vi "Helper SubVI - Fusion Method.vi"(6 "method":u16(ring)=2 items=["Max", "Min", "Mean", "Image 1", "Image 2"], 9 "Coef 2":i32[][](array[numeric]), 11 "Coef 1":i32[][](array[numeric])) -> (3 "Fusion Coef":i32[][](array[numeric]))   [LabVIEW 2023]
doc: "Merges the input coefficients."
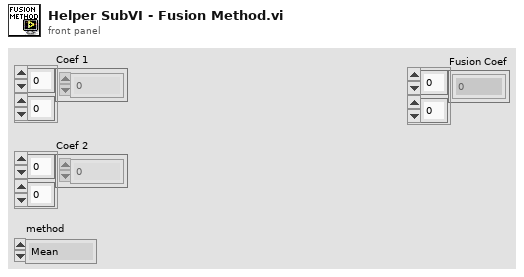
[diagram p1: front panel]
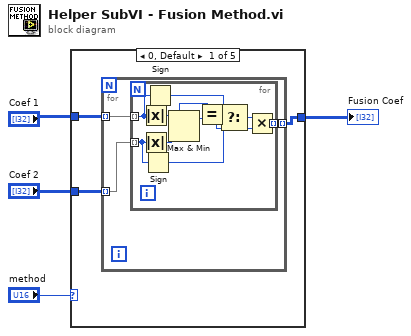
[diagram p0: block diagram]
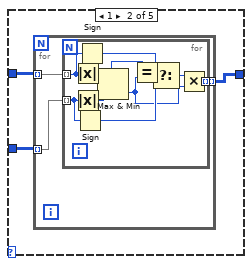
[diagram p2: hidden frame]
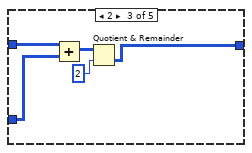
[diagram p3: hidden frame]
diagram:
  n1 = case shown="0, Default" "method" {
    tunnel: "Coef 1" -> [w7 w23 w41 w42 _]
    tunnel: "Coef 2" -> [w6 w22 w40 _ w43]
    tunnel: [w5 w21 w37 w42 w43] -> w1
    frame 0, Default {
      n2 = for {
        tunnel: w7 -> [w10] mode=indexing
        tunnel: w6 -> [w9] mode=indexing
        tunnel: [w8] -> w5 mode=indexing
        n3 = for {
          tunnel: w10 -> [w18] mode=indexing
          tunnel: w9 -> [w19] mode=indexing
          tunnel: [w11] -> w8 mode=indexing
          n4 = Absolute Value(x=w18) -> (abs(x)=w17:i32)
          n5 = Absolute Value(x=w19) -> (abs(x)=w20:i32)
          n6 = Sign(1:w19) -> (0:w14:i32)
          n7 = Sign(1:w18) -> (0:w15:i32)
          n8 = Max & Min(x=w17, y=w20) -> (max(x,y)=w12:i32)  [unwired: 1 out]
          n9 = Equal?(x=w17, y=w12) -> (x = y?=w16:bool)
          n10 = Select(t=w15, s=w16, f=w14) -> (s? t:f=w13:i32)
          n11 = Multiply(x=w13, y=w12) -> (x*y=w11:i32)
        }
      }
    }
    frame 1 {
      n12 = for {
        tunnel: w23 -> [w26] mode=indexing
        tunnel: w22 -> [w25] mode=indexing
        tunnel: [w24] -> w21 mode=indexing
        n13 = for {
          tunnel: w26 -> [w34] mode=indexing
          tunnel: w25 -> [w35] mode=indexing
          tunnel: [w28] -> w24 mode=indexing
          n14 = Absolute Value(x=w34) -> (abs(x)=w33:i32)
          n15 = Absolute Value(x=w35) -> (abs(x)=w36:i32)
          n16 = Sign(1:w35) -> (0:w30:i32)
          n17 = Sign(1:w34) -> (0:w31:i32)
          n18 = Max & Min(x=w33, y=w36) -> (min(x,y)=w27:i32)  [unwired: 1 out]
          n19 = Equal?(x=w33, y=w27) -> (x = y?=w32:bool)
          n20 = Select(t=w31, s=w32, f=w30) -> (s? t:f=w29:i32)
          n21 = Multiply(x=w29, y=w27) -> (x*y=w28:i32)
        }
      }
    }
    frame 2 {
      n22 = Add(x=w41, y=w40) -> (x+y=w39:i32[][])
      n23 = Quotient & Remainder(x=w39, y=2) -> (floor(x/y)=w37:i32[][])  [unwired: 1 out]
    }
    frame 3 {
    }
    frame 4 {
    }
  }
  "Fusion Coef" <- w1
